vi "aa_read_func.vi"(5 "Aardvark Handle":i32 min=0, 6 "No Stop? (False)":bool, 7 "Address (0x50)":u16=80 max=1023 format="%.0x", 8 "error in (no error)":errorcluster, 9 "Combined Format? (False)":bool, 10 "10-bit Addressing? (False)":bool, 11 "Num Bytes to Fetch (64)":u16=64 min=1) -> (0 "error out":errorcluster, 1 "Incoming Data":u8[](array[numeric]) format="%.0x", 2 "Status":i32, 3 "dup Aardvark Handle":i32)   [LabVIEW 2014]
uses:
  aardvark.dll
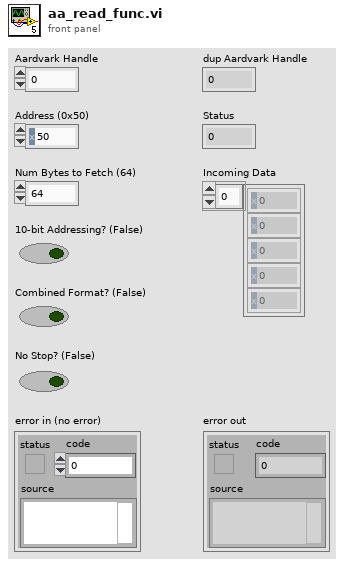
[diagram p1: front panel]
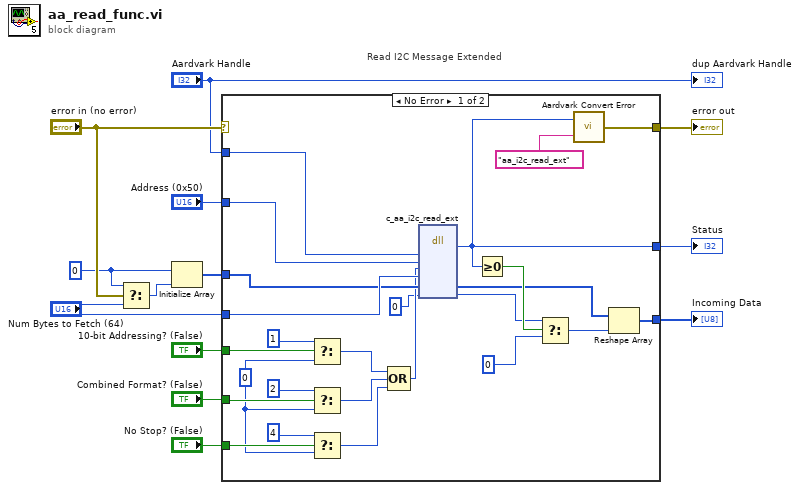
[diagram p0: block diagram]
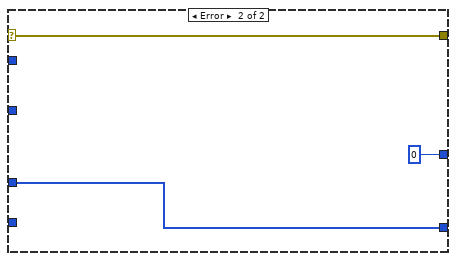
[diagram p2: hidden frame]
diagram:
  w5 = u8 0
  # "Read I2C Message Extended"
  n1 = Select(t=w5, s="error in (no error)", f="Num Bytes to Fetch (64)") -> (s? t:f=w4:u16)
  n2 = Initialize Array(w5, w4) -> (w7:u8[])
  n3 = case shown="No Error" "error in (no error)" {
    selector: "error in (no error)" -> [_ w41]
    tunnel: [w37 w41] -> w1
    tunnel: "Aardvark Handle" -> [w36 _]
    tunnel: [w31 w40] -> w3
    tunnel: w7 -> [w20 w40]
    tunnel: "Num Bytes to Fetch (64)" -> [w21 _]
    tunnel: "Address (0x50)" -> [w35 _]
    tunnel: "10-bit Addressing? (False)" -> [w30 _]
    tunnel: "Combined Format? (False)" -> [w29 _]
    tunnel: "No Stop? (False)" -> [w28 _]
    tunnel: [w15 0] -> w13
    frame No Error {
      w14 = 0
      n4 = Select(t=1, s=w30, f=w14) -> (s? t:f=w24:i32)
      n5 = Select(t=2, s=w29, f=w14) -> (s? t:f=w23:i32)
      n6 = Select(t=4, s=w28, f=w14) -> (s? t:f=w22:i32)
      n7 = Compound Arithmetic op=OR(w24, w23, w22) -> (w19:i32)
      n8 = dll-call lib="aardvark.*" fn="c_aa_i2c_read_ext"("aardvark"=w36, "slave_addr"=w35, "flags"=w19, "num_bytes"=w21, "data_in"=w20, "num_read"=u16 0) -> (w15:i32, "data_in"=w18:u8[], "num_read"=w16:u16)  [unwired: 7 in, 2 out]
      n9 = Greater Or Equal To 0?(x=w15) -> (x >= 0?=w34:bool)
      n10 = Select(t=w16, s=w34, f=0) -> (s? t:f=w32:i32)
      n11 = call <instrlib>:"Aardvark Convert Error.vi"("Source"="aa_i2c_read_ext", "Error Code"=w15) -> ("error out"=w37:errorcluster)
      n12 = Reshape Array(w18, w32) -> (w31:u8[])
    }
    frame Error {
    }
  }
  "error out" <- w1
  "Incoming Data" <- w3
  "Status" <- w13
  "dup Aardvark Handle" <- "Aardvark Handle"
